vi "4Pi Dual DM - Format Voltage Array.vi"(7 "Pixel Level (-1 to 1)":dbl[](array[numeric])) -> (4 "Voltage Array (Volts)":dbl[](array[numeric]), 15 "Pixel Map":dbl[][](array[numeric]))   [LabVIEW 2016]
uses:
  <vilib>/Analysis/baseanly.llb/Mean (DBL).vi
  <vilib>/Analysis/NI_AALBase.lvlib
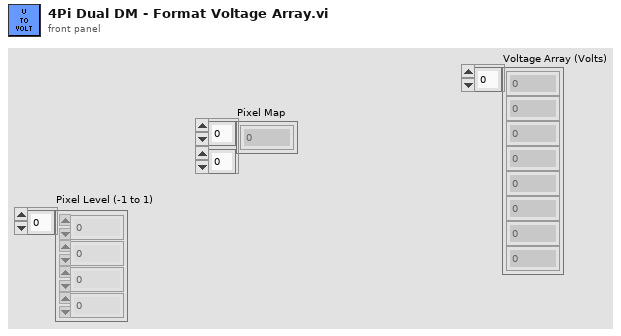
[diagram p1: front panel]
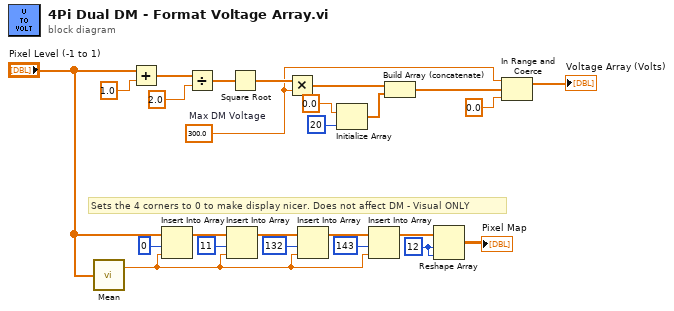
[diagram p0: block diagram]
diagram:
  w1 = 300.0  # Max DM Voltage
  w18 = 12 ("dimension size")
  # "Sets the 4 corners to 0 to make display nicer. Does not affect DM - Visual ONLY"
  n1 = call-poly <vilib>:"Mean.vi"("X"="Pixel Level (-1 to 1)") -> ("mean"=w15:dbl)  [unwired: 1 out]
  n2 = Add(x="Pixel Level (-1 to 1)", y=1.0) -> (x+y=w10:dbl[])
  n3 = Insert Into Array(array="Pixel Level (-1 to 1)", index=0, new element=w15) -> (w23:dbl[])
  n4 = Divide(x=w10, y=2.0) -> (x/y=w8:dbl[])
  n5 = Insert Into Array(array=w23, index=11, new element=w15) -> (w21:dbl[])
  n6 = Square Root(x=w8) -> (sqrt(x)=w7:dbl[])
  n7 = Multiply(x=w7, y=w1) -> (x*y=w6:dbl[])
  n8 = Insert Into Array(array=w21, index=132, new element=w15) -> (w19:dbl[])
  n9 = Initialize Array(0.0 ("element"), 20 ("dimension size")) -> (w12:dbl[])
  n10 = Insert Into Array(array=w19, index=143, new element=w15) -> (w17:dbl[])
  n11 = Build Array (concatenate)(w6, w12) -> (w2:dbl[])
  n12 = Reshape Array(w17, w18, w18) -> (→"Pixel Map":dbl[][])
  n13 = In Range and Coerce(upper limit=w1, x=w2, lower limit=0.0) -> (coerced(x)=→"Voltage Array (Volts)":dbl[])  [unwired: 1 out]
